vi "Shorten String.vi"(7 "max lenght (29)":i32=29, 11 "string in":string) -> (3 "string out":string)   [LabVIEW 2017]
doc: "Shortens the string so that it fits in the frame."
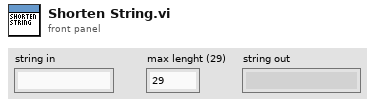
[diagram p1: front panel]
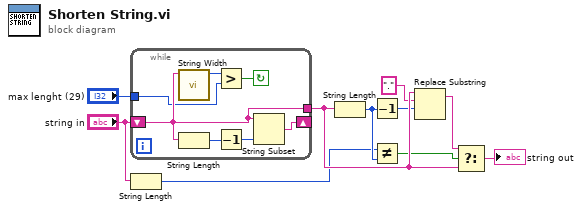
[diagram p0: block diagram]
diagram:
  n1 = while {
    shift-right: [w16] -> _
    shift-left: "string in" -> [w12]
    tunnel: [w12] -> w7
    tunnel: "max lenght (29)" -> [w11]
    stop <- w13 continue-if-true
    n2 = call "String Width.vi"("string"=w12) -> ("string width"=w17:i32)  [unwired: 10 in]
    n3 = String Length(string=w12) -> (length=w15:i32)
    n4 = Greater?(x=w17, y=w11) -> (0:w13:bool)
    n5 = Decrement(x=w15) -> (x-1=w14:i32)
    n6 = String Subset(string=w12, length (rest)=w14) -> (substring=w16:string)  [unwired: 1 in]
  }
  n7 = String Length(string="string in") -> (length=w2:i32)
  n8 = String Length(string=w7) -> (length=w3:i32)
  n9 = Decrement(x=w3) -> (x-1=w4:i32)
  n10 = Not Equal?(x=w2, y=w3) -> (x != y?=w5:bool)
  n11 = Replace Substring(3:w4, 4:"." ("substring (\"\")"), 5:w7) -> (1:w6:string)  [unwired: 1 in, 1 out]
  n12 = Select(t=w6, s=w5, f=w7) -> (s? t:f=→"string out":string)
